vi "Draw Data.vi"(7 "draw options":T3={"Background Color"=16777215, "Grid Color"=13816530, "Angle Units"=enum."Radians", "Draw Solid Background"=TRUE, "Draw Grid"=TRUE, "Grid Spacing"=1.0, "AutoScale"=TRUE, "Fit to Radius"=1.0, "data row options"=[]}, 9 "scaling info":T2={"pixels per unit"=1.0, "fit radius (units)"=1.0, "center point (pixels)"={"x"=0, "y"=0}}, 10 "cartesian data":T1, 11 "picture in":picture) -> (3 "picture out":picture)   [LabVIEW 2017, in "NI_Robotics_2D Rangefinder Picture.lvlib"]
uses:
  <vilib>/robotics/Controls/2D Rangefinder/2D Rangefinder Picture/NI_Robotics_2D Rangefinder Picture.lvlib
  <vilib>/robotics/Controls/2D Rangefinder/2D Rangefinder Picture/Draw Options.ctl
  <vilib>/robotics/Controls/Utilities/Angle Units.ctl
  <vilib>/robotics/Controls/2D Rangefinder/2D Rangefinder Picture/Data Row Options.ctl
  <vilib>/robotics/Controls/2D Rangefinder/2D Rangefinder Picture/Scaling Info.ctl
  <vilib>/robotics/Controls/2D Rangefinder/2D Rangefinder Picture/Cartesian Data.ctl
  <vilib>/robotics/Controls/Utilities/NI_Robotics_Control Utilities.lvlib
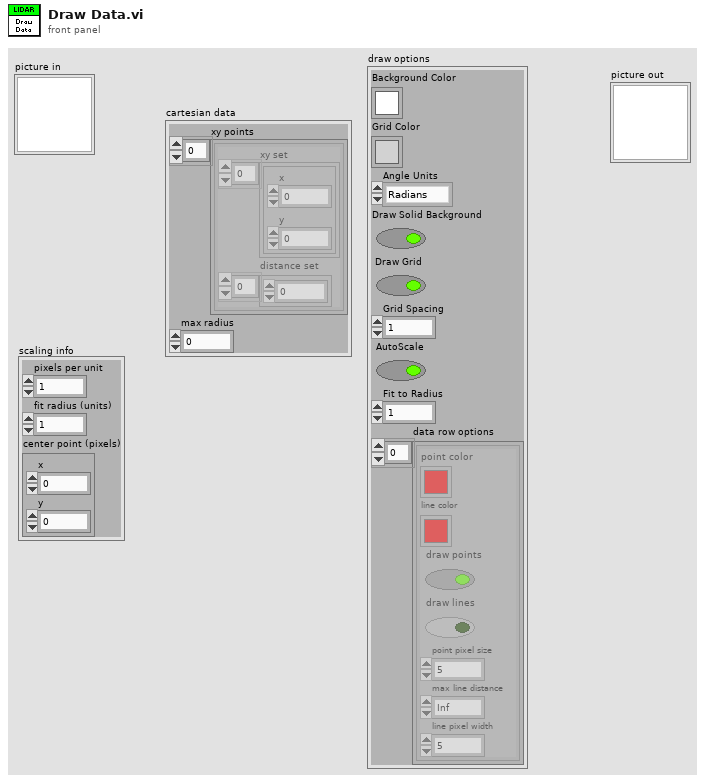
[diagram p1: front panel]
types:
  T1 = typedef "NI_Robotics_2D Rangefinder Picture.lvlib/Cartesian Data.ctl" = cluster{"xy points":cluster{"xy set":cluster{"x":dbl, "y":dbl}[], "distance set":dbl[]}[], "max radius":dbl}
  T2 = typedef "NI_Robotics_2D Rangefinder Picture.lvlib/Scaling Info.ctl" = cluster{"pixels per unit":dbl, "fit radius (units)":dbl, "center point (pixels)":cluster{"x":i16, "y":i16}}
  T3 = typedef "NI_Robotics_2D Rangefinder Picture.lvlib/Draw Options.ctl" = cluster{"Background Color":u32, "Grid Color":u32, "Angle Units":T4, "Draw Solid Background":bool, "Draw Grid":bool, "Grid Spacing":dbl, "AutoScale":bool, "Fit to Radius":dbl, "data row options":T5[]}
  T4 = typedef "NI_Robotics_Control Utilities.lvlib/Angle Units.ctl" = enum16{"Radians", "Degrees"}
  T5 = typedef "NI_Robotics_2D Rangefinder Picture.lvlib/Data Row Options.ctl" = cluster{"point color":u32, "line color":u32, "draw points":bool, "draw lines":bool, "point pixel size":u16, "max line distance":dbl, "line pixel width":u16}
  T6 = cluster{"xy set":cluster{"x":dbl, "y":dbl}[], "distance set":dbl[]}[]
  T7 = cluster{"Width":u16, "Style":enum32{"Solid", "Dash", "Dot", "DashDot", "DashDotDot"}}
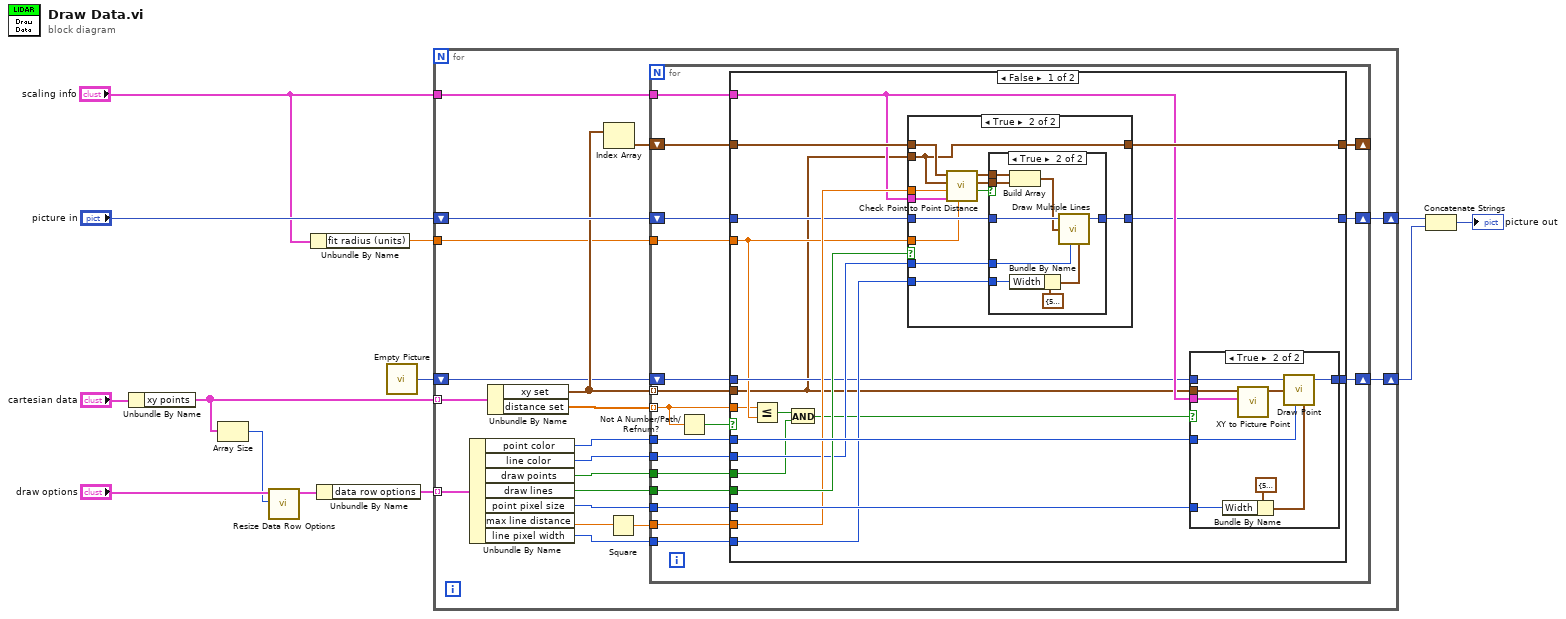
[diagram p0: block diagram]
diagram:
  n1 = Unbundle By Name("cartesian data") -> ("xy points"=w10:T6)
  n2 = Array Size(array=w10) -> (size(s)=w7:i32)
  n3 = call <vilib>:"Resize Data Row Options.vi"("number of data rows (1)"=w7, "draw options in"="draw options") -> ("draw options out"=w8:T3)  [unwired: 9 in]
  n4 = Unbundle By Name("scaling info") -> ("fit radius (units)"=w1:dbl)
  n5 = Unbundle By Name(w8) -> ("data row options"=w11:T5[])
  n6 = call "Empty Picture"() -> ("empty picture"=w6:picture)
  n7 = for {
    tunnel: w10 -> [w32] mode=indexing
    shift-right: [w30] -> w4
    shift-left: "picture in" -> [w31]
    tunnel: "scaling info" -> [w29]
    tunnel: w11 -> [w26] mode=indexing
    shift-right: [w16] -> w5
    shift-left: w6 -> [w17]
    tunnel: w1 -> [w14]
    n8 = Unbundle By Name(w26) -> ("point color"=w25:u32, "line color"=w24:u32, "draw points"=w23:bool, "draw lines"=w22:bool, "point pixel size"=w21:u16, "max line distance"=w19:dbl, "line pixel width"=w20:u16)
    n9 = Unbundle By Name(w32) -> ("xy set"=w28:cluster{"x":dbl, "y":dbl}[], "distance set"=w15:dbl[])
    n10 = Index Array(array=w28) -> (element=w27:cluster{"x":dbl, "y":dbl})  [unwired: 1 in]
    n11 = Square(x=w19) -> (x^2=w18:dbl)
    n12 = for {
      tunnel: w28 -> [w35] mode=indexing
      shift-right: [w40] -> w30
      shift-left: w31 -> [w41]
      tunnel: w29 -> [w44]
      tunnel: w25 -> [w50]
      tunnel: w24 -> [w43]
      tunnel: w21 -> [w49]
      shift-right: [w46] -> _
      shift-left: w27 -> [w47]
      tunnel: w23 -> [w36]
      tunnel: w22 -> [w48]
      tunnel: w18 -> [w45]
      tunnel: w20 -> [w42]
      shift-right: [w38] -> w16
      shift-left: w17 -> [w39]
      tunnel: w15 -> [w34] mode=indexing
      tunnel: w14 -> [w37]
      n13 = Not A Number/Path/Refnum?(number/path/refnum=w34) -> (NaN/Path/Refnum?=w33:bool)
      n14 = case shown="False" w33 {
        tunnel: w50 -> [w69 _]
        tunnel: w49 -> [w68 _]
        tunnel: w48 -> [w67 _]
        tunnel: w47 -> [w66 w106]
        tunnel: [w65 w106] -> w46
        tunnel: w45 -> [w64 _]
        tunnel: w44 -> [w63 _]
        tunnel: w43 -> [w62 _]
        tunnel: w42 -> [w61 _]
        tunnel: w41 -> [w60 w105]
        tunnel: [w59 w105] -> w40
        tunnel: w39 -> [w58 w104]
        tunnel: [w57 w104] -> w38
        tunnel: w37 -> [w56 _]
        tunnel: w36 -> [w54 _]
        tunnel: w35 -> [w52 _]
        tunnel: w34 -> [w51 _]
        frame False {
          n15 = Less Or Equal?(x=w51, y=w56) -> (x <= y?=w55:bool)
          n16 = And(x=w55, y=w54) -> (x .and. y?=w53:bool)
          n17 = case shown="True" w67 {
            tunnel: w60 -> [w71 w76]
            tunnel: [w71 w75] -> w59
            tunnel: w66 -> [w70 w83]
            tunnel: w52 -> [_ w82]
            tunnel: [w70 w82] -> w65
            tunnel: w64 -> [_ w81]
            tunnel: w63 -> [_ w80]
            tunnel: w62 -> [_ w74]
            tunnel: w61 -> [_ w73]
            tunnel: w56 -> [_ w72]
            frame False {
            }
            frame True {
              n18 = call <vilib>:"Check Point to Point Distance.vi"("fit radius"=w72, "scaling info"=w80, "max dist squared"=w81, "P2 (units)"=w82, "P1 (units)"=w83) -> ("valid?"=w79:bool, "P2 (pixels)"=w77:cluster{"x":i16, "y":i16}, "P1 (pixels)"=w78:cluster{"x":i16, "y":i16})  [unwired: 4 in]
              n19 = case shown="True" w79 {
                tunnel: w78 -> [_ w87]
                tunnel: w77 -> [_ w86]
                tunnel: w76 -> [w84 w93]
                tunnel: [w84 w92] -> w75
                tunnel: w74 -> [_ w91]
                tunnel: w73 -> [_ w88]
                frame False {
                }
                frame True {
                  n20 = Build Array(w87, w86) -> (w85:cluster{"x":i16, "y":i16}[])
                  n21 = Bundle By Name(cluster=T7 {"Width"=5, "Style"=enum."Solid"} ("pen"), "Width"=w88) -> (w89:T7)
                  n22 = call <vilib>:"Draw Multiple Lines.vi"("picture"=w93, "line endpoints"=w85, "color(black)"=w91, "pen"=w89) -> ("new picture"=w92:picture)  [unwired: 5 in]
                }
              }
            }
          }
          n23 = case shown="True" w53 {
            tunnel: w52 -> [_ w103]
            tunnel: w63 -> [_ w102]
            tunnel: w58 -> [w94 w101]
            tunnel: [w94 w100] -> w57
            tunnel: w69 -> [_ w98]
            tunnel: w68 -> [_ w96]
            frame False {
            }
            frame True {
              n24 = Bundle By Name(cluster=T7 {"Width"=5, "Style"=enum."Solid"} ("pen"), "Width"=w96) -> (w95:T7)
              n25 = call <vilib>:"XY to Picture Point.vi"("scaling info"=w102, "xy point (units)"=w103) -> ("xy point (pixels)"=w99:cluster{"x":i16, "y":i16})  [unwired: 9 in]
              n26 = call <vilib>:"Draw Point.vi"("picture"=w101, "point(x,y)"=w99, "color(black)"=w98, "pen"=w95) -> ("new picture"=w100:picture)  [unwired: 5 in]
            }
          }
        }
        frame True {
        }
      }
    }
  }
  n27 = Concatenate Strings(w4, w5) -> (→"picture out":picture)
